vi "Features_SpecPage.vi"(10 "Spec Page Interface":T1, 11 "MetaDataObj in":refnum<class "MetaDataObj.lvclass">) -> (3 "MetaDataObj out":refnum<class "MetaDataObj.lvclass">)   [LabVIEW 2013, in "editorscriptingobjectBasicExec.lvclass"]
uses:
  editorscriptingobjectBasicExec.lvclass
  <resource>/dialog/NewProjectWizard/Spec Page Interface.ctl
  <resource>/dialog/NewProjectWizard/MetaDataObj/MetaDataObj.lvclass
  <resource>/dialog/NewProjectWizard/MetaDataObj/MetaDataObj.lvclass/MetaDataObj.ctl
  <resource>/dialog/NewProjectWizard/MetaDataObj/Accessors/Write Project Name.vi
  <resource>/dialog/NewProjectWizard/MetaDataObj/Accessors/Write Project Root.vi
  <resource>/dialog/NewProjectWizard/MetaDataObj/Accessors/Write File Prefix.vi
panel:
  in  "Project Name":string
  in  "Project Root":path
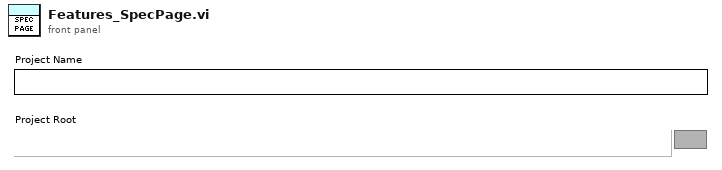
[diagram p1: front panel]
types:
  T1 = typedef "Spec Page Interface.ctl" = cluster{"\"Tab Forward To\" Refnum":refnum<vi>, "\"Tab Backward To\" Refnum":refnum<vi>, "Errors":refnum<user-event>, "Quit":refnum<user-event>}
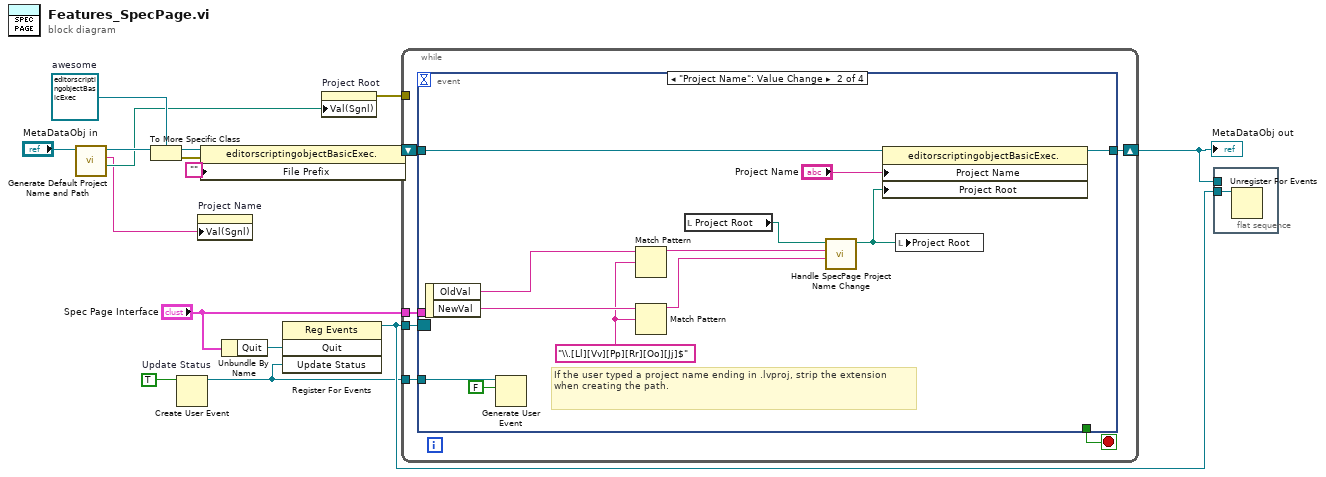
[diagram p0: block diagram]
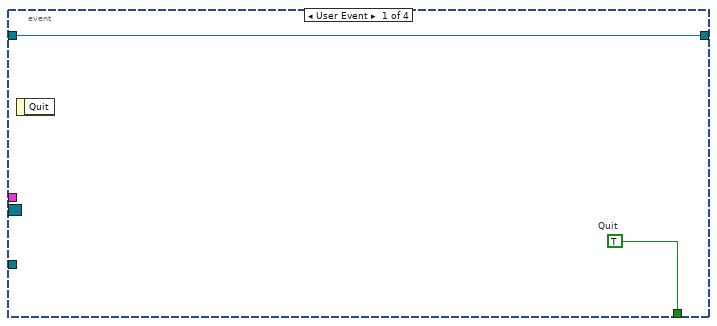
[diagram p2: hidden frame]
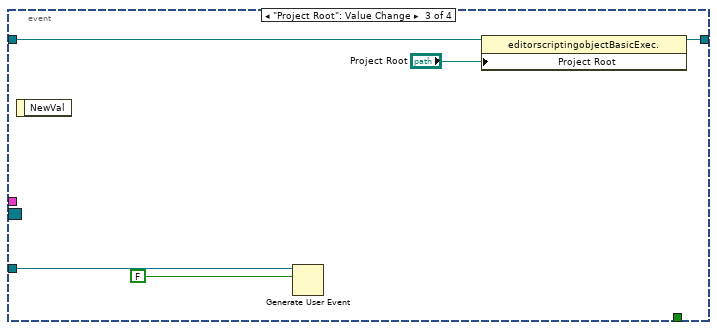
[diagram p3: hidden frame]
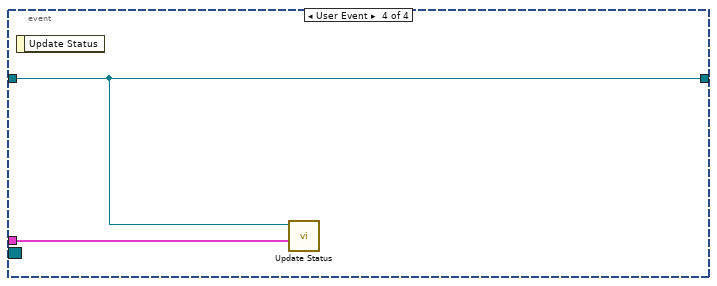
[diagram p4: hidden frame]
diagram:
  w10 = TRUE  # Update Status
  w11 = refnum<class "editorscriptingobjectBasicExec.lvclass"> refnum  # awesome
  n1 = call <resource>:"Generate Default Project Name and Path.vi"("DNL_MetaDataObj in"="MetaDataObj in") -> ("Project Root"=w3:path, "Project Name"=w1:string, "DNL_MetaDataObj out"=w4:refnum<class "MetaDataObj.lvclass">)  [unwired: 8 in]
  n2 = To More Specific Class(target class=w11, reference=w4) -> (specific class reference=w13:refnum<class "editorscriptingobjectBasicExec.lvclass">, error out=w12:errorcluster)  [unwired: 1 in]
  n3 = Create User Event(user event datatype=w10) -> (user event=w7:refnum<user-event>)  [unwired: 1 in, 1 out]
  n4 = property on="Project Name" class="Str"("Val(Sgnl)"=w1) -> ()  [unwired: 2 in, 2 out]
  n5 = property class="editorscriptingobjectBasicExec."(reference=w13, error in=w12, "File Prefix"="") -> (reference out=w9:refnum<class "editorscriptingobjectBasicExec.lvclass">)  [unwired: 1 out]
  n6 = Unbundle By Name("Spec Page Interface") -> ("Quit"=w16:refnum<user-event>)
  n7 = register-events(w16, w7) -> (reference out=w15:refnum<event-registration>)  [unwired: 2 in, 1 out]
  n8 = property on="Project Root" class="Path"("Val(Sgnl)"=w3) -> (error out=w8:errorcluster)  [unwired: 2 in, 1 out]
  n9 = while {
    tunnel: "Spec Page Interface" -> [w21]
    shift-right: [w19] -> w2
    shift-left: w9 -> [w18]
    tunnel: w15 -> [w20]
    tunnel: w8 -> [_]
    tunnel: w7 -> [w17]
    stop <- w22 stop-if-true
    n10 = event shown="[1] \"Project Name\": Value Change" {
      selector: w20 -> [_ _ _ _]
      dyn-events: _ -> [_ _ _ _]
      timeout: _ -> [_ _ _ _]
      tunnel: w21 -> [_ _ _ w42]
      tunnel: [w24 _ _ _] -> w22
      tunnel: [w23 w36 w40 w43] -> w19
      tunnel: w18 -> [w23 w33 w41 w43]
      tunnel: w17 -> [_ w35 w39 _]
      event User Event {
        w24 = TRUE  # Quit
        n11 = event-data() -> ()  [unwired: 1 in, 1 out]
      }
      event "Project Name": Value Change {
        w28 = "\\.[Ll][Vv][Pp][Rr][Oo][Jj]$" ("regular expression")
        # "If the user typed a project name ending in .lvproj, strip the extension when creating the path."
        n12 = event-data() -> ("OldVal"=w30:string, "NewVal"=w29:string)  [unwired: 1 in]
        n13 = Generate User Event(user event=w35, event data cluster=FALSE ("Update Status")) -> ()  [unwired: 2 in, 2 out]
        n14 = Match Pattern(string=w30, regular expression=w28) -> (before substring=w27:string)  [unwired: 1 in, 3 out]
        n15 = Match Pattern(string=w29, regular expression=w28) -> (before substring=w26:string)  [unwired: 1 in, 3 out]
        n16 = local read "Project Root"() -> (w32:path)
        n17 = call <resource>:"Handle SpecPage Project Name Change.vi"("Project Name New Value"=w26, "Project Name Old Value"=w27, "Project Root in"=w32) -> ("Project Root out"=w31:path)  [unwired: 8 in]
        n18 = property class="editorscriptingobjectBasicExec."(reference=w33, "Project Name"="Project Name", "Project Root"=w31) -> (reference out=w36:refnum<class "editorscriptingobjectBasicExec.lvclass">)  [unwired: 1 in, 1 out]
        n19 = local write "Project Root"(w31) -> ()
      }
      event "Project Root": Value Change {
        n20 = event-data() -> ()  [unwired: 1 in, 1 out]
        n21 = Generate User Event(user event=w39, event data cluster=FALSE ("Update Status")) -> ()  [unwired: 2 in, 2 out]
        n22 = property class="editorscriptingobjectBasicExec."(reference=w41, "Project Root"="Project Root") -> (reference out=w40:refnum<class "editorscriptingobjectBasicExec.lvclass">)  [unwired: 1 in, 1 out]
      }
      event User Event {
        n23 = event-data() -> ()  [unwired: 1 in, 1 out]
        n24 = call "Update Status.vi"("Spec Page Interface"=w42, "TwoTasksMetaDataObj in"=w43) -> ()  [unwired: 10 in]
      }
    }
  }
  "MetaDataObj out" <- w2
  n25 = flat-sequence {
    tunnel: w15 -> [w44]
    tunnel: w2 -> [_]
    frame #0 {
      n26 = Unregister For Events(event registration refnum=w44) -> ()  [unwired: 1 in, 1 out]
    }
  }
